vi "GetCommandLinePars.vi"(0 "Command line array":string[](array[string])) -> (1 "Server":string, 2 "Port":i32=2402, 3 "AzCamToolParFile":path, 4 "Found?":bool)   [LabVIEW 2014]
uses:
  globals/AzCamGlobals.vi
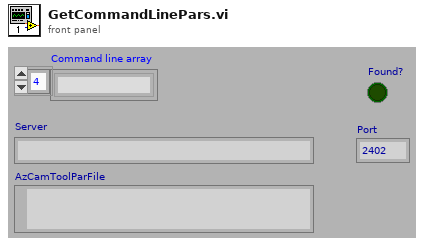
[diagram p1: front panel]
types:
  T1 = enum32{"invalid app kind", "Development System", "Run Time System", "Student Edition", "Embedded LabVIEW", "Evaluation", "Custom"}
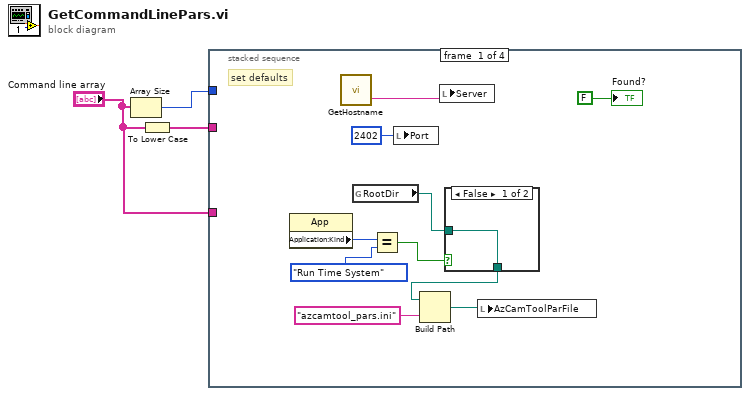
[diagram p0: block diagram]
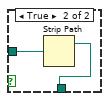
[diagram p2: hidden frame]
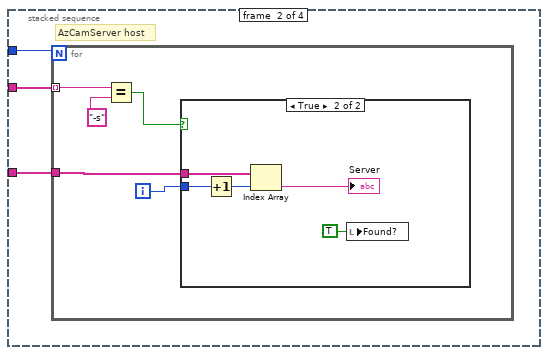
[diagram p3: hidden frame]
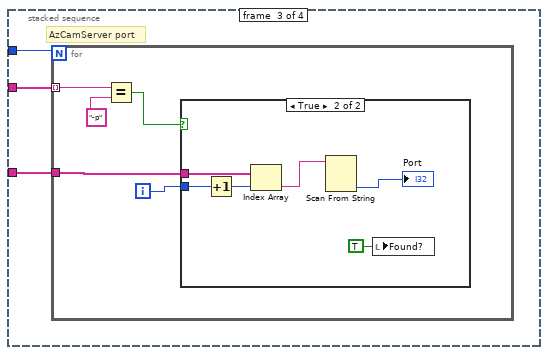
[diagram p5: hidden frame]
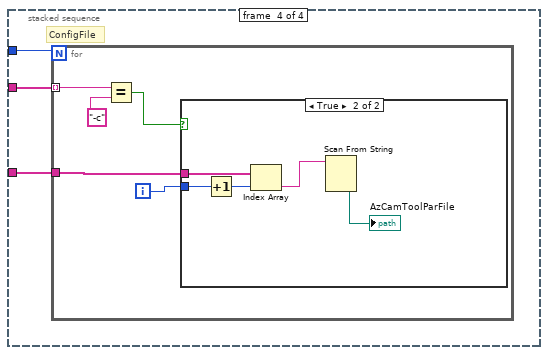
[diagram p7: hidden frame]
diagram:
  n1 = Array Size(array="Command line array") -> (size(s)=w3:i32)
  n2 = To Lower Case(string="Command line array") -> (all lower case string=w1:string[])
  n3 = stacked-sequence {
    tunnel: w3 -> [_ w19 w32 w46]
    tunnel: "Command line array" -> [_ w17 w30 w44]
    tunnel: w1 -> [_ w18 w31 w45]
    frame #0 {
      # "set defaults"
      n4 = property class="App"() -> ("Application:Kind"=w7:T1)  [unwired: 2 in, 2 out]
      n5 = call "GetHostname.vi"() -> ("Name"=w12:string)  [unwired: 1 in, 1 out]
      n6 = global read "AzCamGlobals.vi" "RootDir"() -> (w10:path)
      n7 = Equal?(x=w7, y=T1."Run Time System" ("Application:Kind")) -> (x = y?=w9:bool)
      n8 = local write "Port"(2402 ("Port")) -> ()
      n9 = local write "Server"(w12) -> ()
      n10 = case shown="False" w9 {
        tunnel: [w14 w15] -> w11
        tunnel: w10 -> [w14 w16]
        frame False {
        }
        frame True {
          n11 = Strip Path(path=w16) -> (stripped path=w15:path)  [unwired: 1 out]
        }
      }
      n12 = Build Path(base path=w11, name or relative path="azcamtool_pars.ini") -> (appended path=w5:path)
      n13 = local write "AzCamToolParFile"(w5) -> ()
      "Found?" <- FALSE ("Found?")
    }
    frame #1 {
      # "AzCamServer host"
      n14 = for {
        N: w19 -> [_]
        tunnel: w18 -> [w22] mode=indexing
        tunnel: w17 -> [w21]
        i -> [w20]
        n15 = Equal?(x=w22, y="-s" ("x")) -> (x = y?=w23:bool)
        n16 = case shown="True" w23 {
          tunnel: w21 -> [_ w28]
          tunnel: w20 -> [_ w27]
          frame False {
          }
          frame True {
            n17 = Increment(x=w27) -> (x+1=w29:i32)
            n18 = Index Array(array=w28, index=w29) -> (element=→"Server":string)
            n19 = local write "Found?"(TRUE ("Found?")) -> ()
          }
        }
      }
    }
    frame #2 {
      # "AzCamServer port"
      n20 = for {
        N: w32 -> [_]
        tunnel: w31 -> [w35] mode=indexing
        tunnel: w30 -> [w34]
        i -> [w33]
        n21 = Equal?(x=w35, y="-p" ("x")) -> (x = y?=w36:bool)
        n22 = case shown="True" w36 {
          tunnel: w34 -> [_ w42]
          tunnel: w33 -> [_ w41]
          frame False {
          }
          frame True {
            n23 = Increment(x=w41) -> (x+1=w43:i32)
            n24 = Index Array(array=w42, index=w43) -> (element=w40:string)
            n25 = Scan From String(input string=w40) -> (output 1=→"Port":i32)  [unwired: 4 in, 3 out]
            n26 = local write "Found?"(TRUE ("Found?")) -> ()
          }
        }
      }
    }
    frame #3 {
      # "ConfigFile"
      n27 = for {
        N: w46 -> [_]
        tunnel: w45 -> [w49] mode=indexing
        tunnel: w44 -> [w48]
        i -> [w47]
        n28 = Equal?(x=w49, y="-c" ("x")) -> (x = y?=w50:bool)
        n29 = case shown="True" w50 {
          tunnel: w48 -> [_ w55]
          tunnel: w47 -> [_ w54]
          frame False {
          }
          frame True {
            n30 = Increment(x=w54) -> (x+1=w56:i32)
            n31 = Index Array(array=w55, index=w56) -> (element=w53:string)
            n32 = Scan From String(input string=w53) -> (output 1=→"AzCamToolParFile":path)  [unwired: 4 in, 3 out]
          }
        }
      }
    }
  }
